vi "Debug.vi"() -> ()   [LabVIEW 2019, in "Globals.lvlib"]
doc: "Global for holding basic debug info when required."
uses:
  Globals.lvlib
panel:
  in  "Audio Transfer Latency (ms)":dbl
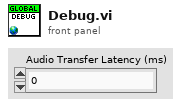
[diagram p1: front panel]
diagram:
